vi "Antenna coordinate ECI.vi"(8 "Antenna altitude":dbl, 9 "Antenna east longitude (°)":dbl, 10 "Antenna latitude (°)":dbl, 11 "tetag (rad)":dbl) -> (2 "Antenna coordinates ECI":T1)   [LabVIEW 2015]
uses:
  <vilib>/Analysis/Matrix/Datatypes/RealMatrix.ctl
  <vilib>/Analysis/Matrix/NI_Matrix.lvlib
panel:
  # "(km)"
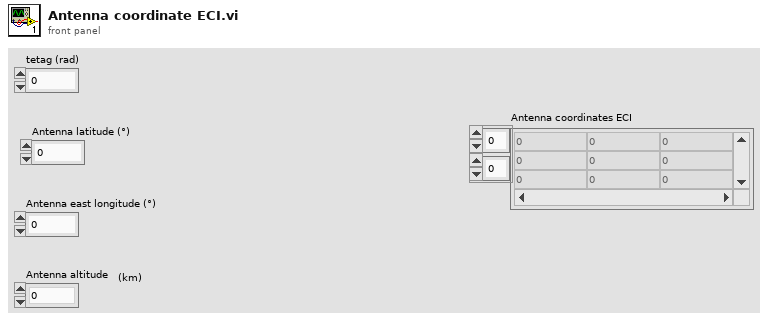
[diagram p1: front panel]
types:
  T1 = typedef "NI_Matrix.lvlib/RealMatrix.ctl" = dbl[][]
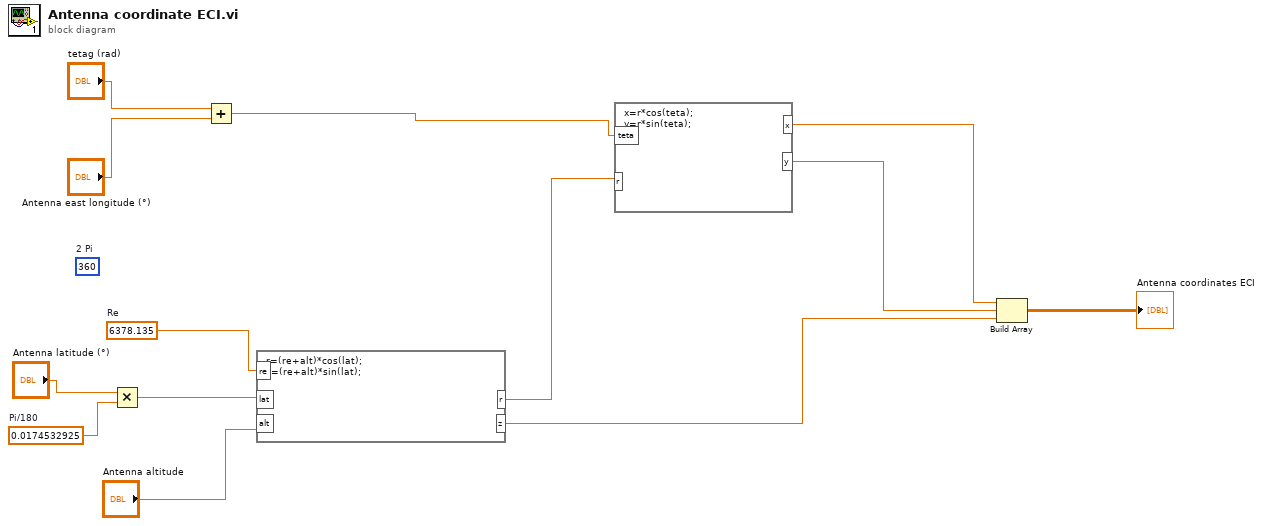
[diagram p0: block diagram]
diagram:
  w7 = 0.0174532925  # Pi/180
  w11 = 6378.135  # Re
  (unwired) 360  # 2 Pi
  n1 = Multiply(x="Antenna latitude (°)", y=w7) -> (x*y=w6:dbl)
  n2 = Add(x="tetag (rad)", y="Antenna east longitude (°)") -> (x+y=w1:dbl)
  n3 = formula code="r=(re+alt)*cos(lat);\nz=(re+alt)*sin(lat);"("re"=w11, "lat"=w6, "alt"="Antenna altitude") -> ("r"=w9:dbl, "z"=w3:dbl)
  n4 = formula code="x=r*cos(teta);\ny=r*sin(teta);"("teta"=w1, "r"=w9) -> ("x"=w5:dbl, "y"=w4:dbl)
  n5 = Build Array(w5, w4, w3) -> (→"Antenna coordinates ECI":T1)
